vi "Is Valid.vi"(8 "error in (no error)":errorcluster, 11 "PrefsDB in":refnum<class "PrefsDB.lvclass">) -> (0 "error out":errorcluster, 2 "Is Valid":bool, 3 "PrefsDB out":refnum<class "PrefsDB.lvclass">)   [LabVIEW 2020, in "User Prefs.lvlib" / "PrefsDB.lvclass"]
uses:
  PrefsDB.lvclass
  PrefsDB.lvclass/PrefsDB.ctl
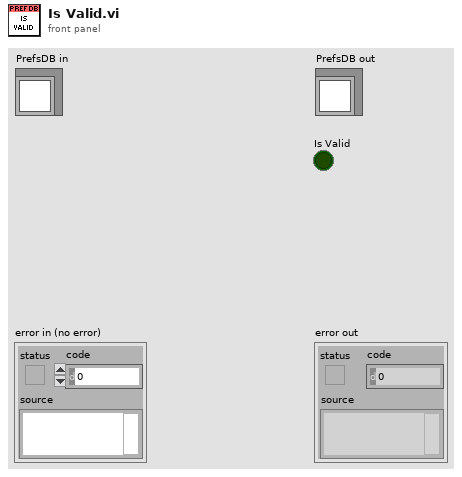
[diagram p1: front panel]
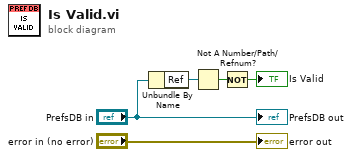
[diagram p0: block diagram]
diagram:
  n1 = Unbundle By Name("PrefsDB in") -> ("Ref"=w3:refnum<data-value>)
  n2 = Not A Number/Path/Refnum?(number/path/refnum=w3) -> (NaN/Path/Refnum?=w2:bool)
  n3 = Not(x=w2) -> (.not. x?=→"Is Valid":bool)
  "error out" <- "error in (no error)"
  "PrefsDB out" <- "PrefsDB in"
